vi "search for matching editor.vi"(11 "LabVIEW Object in":refnum<class>) -> (3 "appended path":path)   [LabVIEW 2013]
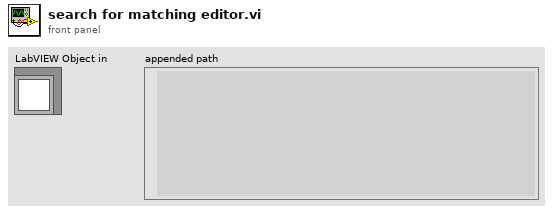
[diagram p1: front panel]
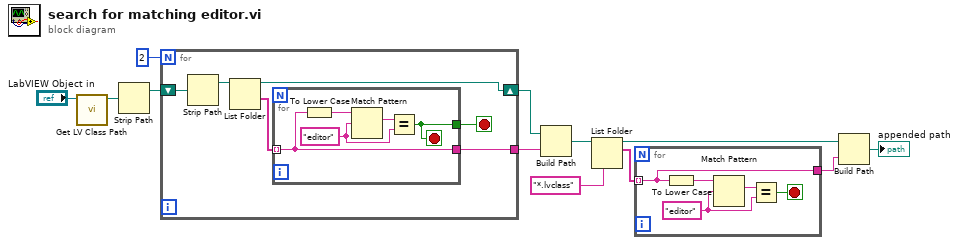
[diagram p0: block diagram]
diagram:
  n1 = call <vilib>:"Get LV Class Path.vi"("object"="LabVIEW Object in") -> ("class path"=w2:path)  [unwired: 9 in, 1 out]
  n2 = Strip Path(path=w2) -> (stripped path=w1:path)  [unwired: 1 out]
  n3 = for {
    N: 2 -> [_]
    tunnel: [w15] -> w5
    shift-right: [w14] -> w4
    shift-left: w1 -> [w18]
    stop <- w13 stop-if-true
    n4 = Strip Path(path=w18) -> (stripped path=w17:path)  [unwired: 1 out]
    n5 = List Folder(path=w17) -> (path out=w14:path, folder names=w16:string[])  [unwired: 3 in, 2 out]
    n6 = for {
      tunnel: w16 -> [w20] mode=indexing
      tunnel: [w20] -> w15
      tunnel: [w19] -> w13
      stop <- w19 stop-if-true
      w21 = "editor" ("regular expression")
      n7 = To Lower Case(string=w20) -> (all lower case string=w23:string)
      n8 = Match Pattern(string=w23, regular expression=w21) -> (match substring=w22:string)  [unwired: 1 in, 3 out]
      n9 = Equal?(x=w22, y=w21) -> (x = y?=w19:bool)
    }
  }
  n10 = Build Path(base path=w4, name or relative path=w5) -> (appended path=w6:path)
  n11 = List Folder(path=w6, pattern="*.lvclass") -> (path out=w10:path, filenames=w8:string[])  [unwired: 2 in, 2 out]
  n12 = for {
    tunnel: w8 -> [w25] mode=indexing
    tunnel: [w25] -> w9
    stop <- w24 stop-if-true
    w26 = "editor" ("regular expression")
    n13 = To Lower Case(string=w25) -> (all lower case string=w28:string)
    n14 = Match Pattern(string=w28, regular expression=w26) -> (match substring=w27:string)  [unwired: 1 in, 3 out]
    n15 = Equal?(x=w27, y=w26) -> (x = y?=w24:bool)
  }
  n16 = Build Path(base path=w10, name or relative path=w9) -> (appended path=→"appended path":path)
